vi "Flancos_3.vi"() -> ()   [LabVIEW 2017]
panel:
  out "Conteo 4":bool
  out "Conteo 3":bool
  out "Conteo 2":bool
  in  "Alarma":bool
  in  "Alarma 2":bool
  in  "Alarma 3":bool
  in  "Alarma 4":bool
  out "Conteo":bool
  in  "Seleccion":bool
  out "Waveform Chart":dbl(graph)
  out "Falling 4":dbl
  out "Rise 4":dbl
  out "Falling 3":dbl
  out "Rise 3":dbl
  out "Falling 2":dbl
  out "Rise 2":dbl
  out "Falling":dbl
  out "Rise":dbl
  in  "stop":bool
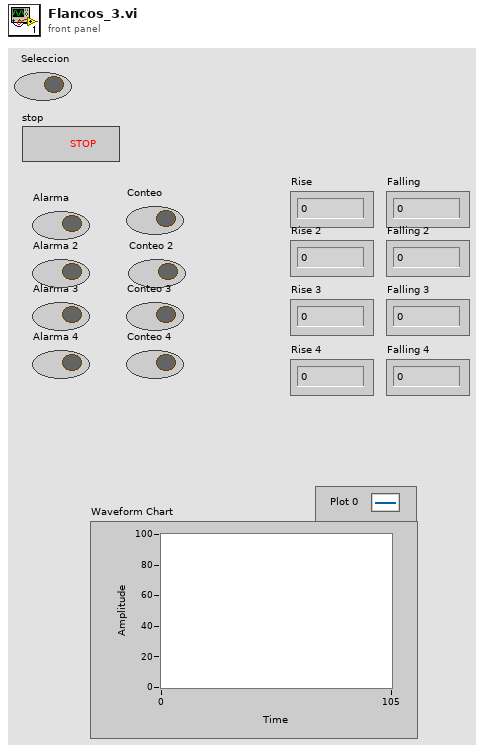
[diagram p1: front panel]
types:
  T1 = cluster{"Cont":i32, "Cont2":i32, "Cont3":i32, "Cont4":i32, "Bajada":i32, "Bajada 2":i32, "Bajada 3":i32, "Bajada 4":i32}
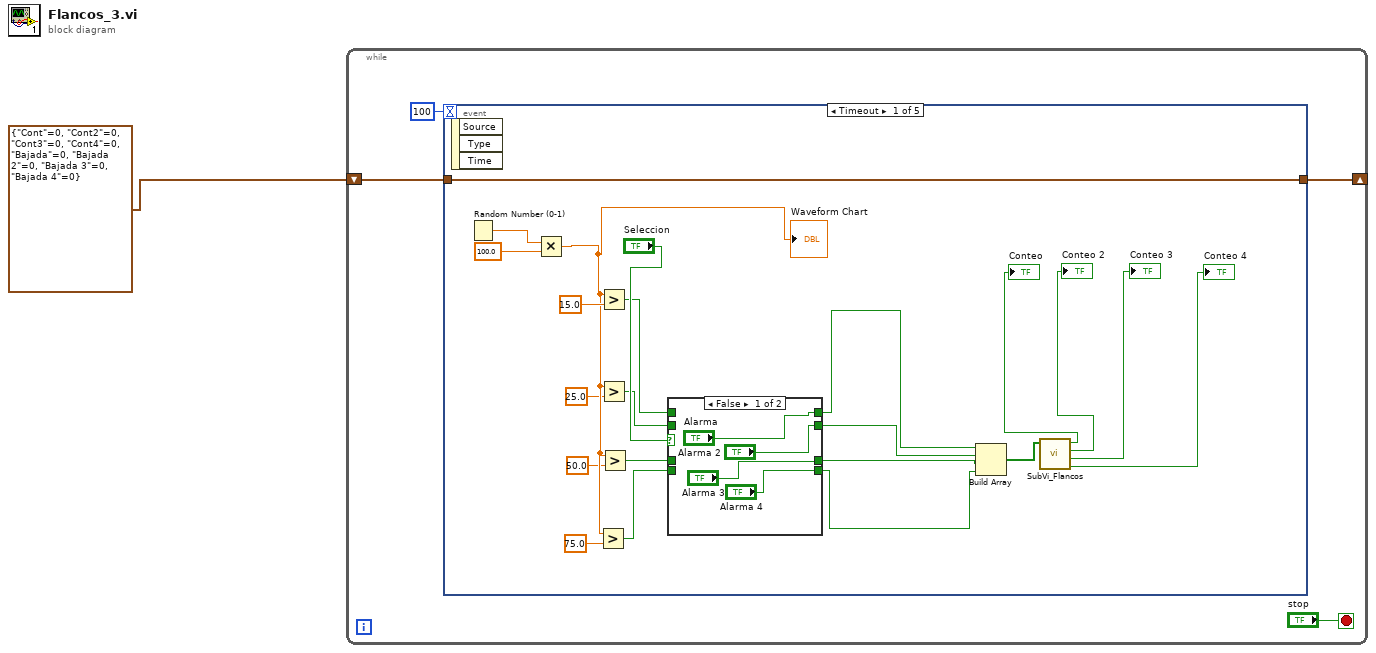
[diagram p0: block diagram]
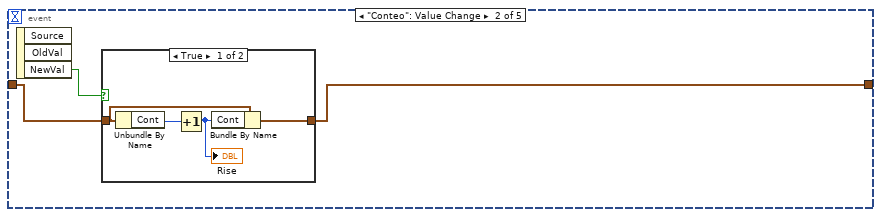
[diagram p3: hidden frame]
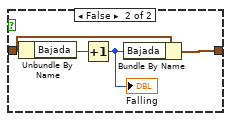
[diagram p4: hidden frame]
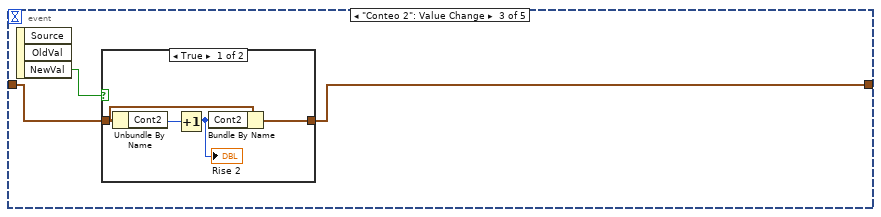
[diagram p5: hidden frame]
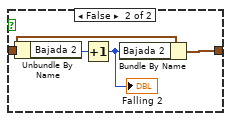
[diagram p6: hidden frame]
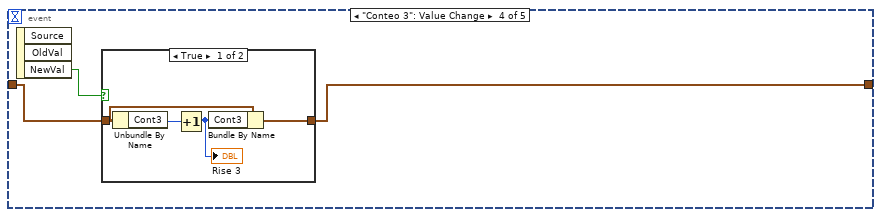
[diagram p7: hidden frame]
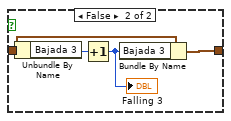
[diagram p8: hidden frame]
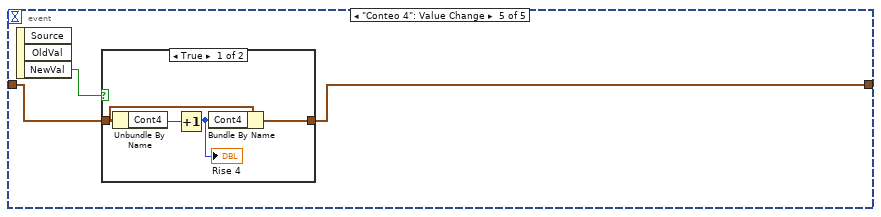
[diagram p9: hidden frame]
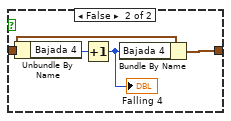
[diagram p10: hidden frame]
diagram:
  n1 = while {
    shift-right: [w3] -> _
    shift-left: T1 {"Cont"=0, "Cont2"=0, "Cont3"=0, "Cont4"=0, "Bajada"=0, "Bajada 2"=0, "Bajada 3"=0, "Bajada 4"=0} -> [w5]
    stop <- "stop" stop-if-true
    n2 = event shown="[0] Timeout" {
      selector: _ -> [_ _ _ _ _]
      dyn-events: _ -> [_ _ _ _ _]
      timeout: 100 -> [_ _ _ _ _]
      tunnel: w5 -> [w27 w38 w49 w60 w71]
      tunnel: [w27 w37 w48 w59 w70] -> w3
      event Timeout {
        n3 = event-data() -> ()  [unwired: 1 in, 3 out]
        n4 = Random Number (0-1)() -> (number: 0 to 1=w26:dbl)
        n5 = Multiply(x=w26, y=100.0) -> (x*y=w23:dbl)
        "Waveform Chart" <- w23
        n6 = Greater?(x=w23, y=75.0) -> (0:w15:bool)
        n7 = Greater?(x=w23, y=15.0) -> (0:w18:bool)
        n8 = Greater?(x=w23, y=25.0) -> (0:w17:bool)
        n9 = Greater?(x=w23, y=50.0) -> (0:w16:bool)
        n10 = case shown="False" "Seleccion" {
          tunnel: w18 -> [_ w35]
          tunnel: w17 -> [_ w34]
          tunnel: w16 -> [_ w33]
          tunnel: w15 -> [_ w32]
          tunnel: ["Alarma" w35] -> w11
          tunnel: ["Alarma 2" w34] -> w12
          tunnel: ["Alarma 3" w33] -> w13
          tunnel: ["Alarma 4" w32] -> w14
          frame False {
          }
          frame True {
          }
        }
        n11 = Build Array(w11, w12, w13, w14) -> (w10:bool[])
        n12 = call "SubVi_Flancos.vi"("Alarmas"=w10) -> ("Conteo 3"=→"Conteo 4":bool, "Conteo 2"=→"Conteo 3":bool, "Conteo 1"=→"Conteo 2":bool, "Conteo"=→"Conteo":bool)  [unwired: 7 in]
      }
      event "Conteo": Value Change {
        n13 = event-data() -> ("NewVal"=w36:bool)  [unwired: 1 in, 2 out]
        n14 = case shown="True" w36 {
          tunnel: w38 -> [w41 w45]
          tunnel: [w40 w44] -> w37
          frame True {
            n15 = Unbundle By Name(w41) -> ("Cont"=w42:i32)
            n16 = Increment(x=w42) -> (x+1=w39:i32)
            "Rise" <- w39
            n17 = Bundle By Name(cluster=w41, "Cont"=w39) -> (w40:T1)
          }
          frame False {
            n18 = Unbundle By Name(w45) -> ("Bajada"=w46:i32)
            n19 = Increment(x=w46) -> (x+1=w43:i32)
            "Falling" <- w43
            n20 = Bundle By Name(cluster=w45, "Bajada"=w43) -> (w44:T1)
          }
        }
      }
      event "Conteo 2": Value Change {
        n21 = event-data() -> ("NewVal"=w47:bool)  [unwired: 1 in, 2 out]
        n22 = case shown="True" w47 {
          tunnel: w49 -> [w52 w56]
          tunnel: [w51 w55] -> w48
          frame True {
            n23 = Unbundle By Name(w52) -> ("Cont2"=w53:i32)
            n24 = Increment(x=w53) -> (x+1=w50:i32)
            "Rise 2" <- w50
            n25 = Bundle By Name(cluster=w52, "Cont2"=w50) -> (w51:T1)
          }
          frame False {
            n26 = Unbundle By Name(w56) -> ("Bajada 2"=w57:i32)
            n27 = Increment(x=w57) -> (x+1=w54:i32)
            "Falling 2" <- w54
            n28 = Bundle By Name(cluster=w56, "Bajada 2"=w54) -> (w55:T1)
          }
        }
      }
      event "Conteo 3": Value Change {
        n29 = event-data() -> ("NewVal"=w58:bool)  [unwired: 1 in, 2 out]
        n30 = case shown="True" w58 {
          tunnel: w60 -> [w63 w67]
          tunnel: [w62 w66] -> w59
          frame True {
            n31 = Unbundle By Name(w63) -> ("Cont3"=w64:i32)
            n32 = Increment(x=w64) -> (x+1=w61:i32)
            "Rise 3" <- w61
            n33 = Bundle By Name(cluster=w63, "Cont3"=w61) -> (w62:T1)
          }
          frame False {
            n34 = Unbundle By Name(w67) -> ("Bajada 3"=w68:i32)
            n35 = Increment(x=w68) -> (x+1=w65:i32)
            "Falling 3" <- w65
            n36 = Bundle By Name(cluster=w67, "Bajada 3"=w65) -> (w66:T1)
          }
        }
      }
      event "Conteo 4": Value Change {
        n37 = event-data() -> ("NewVal"=w69:bool)  [unwired: 1 in, 2 out]
        n38 = case shown="True" w69 {
          tunnel: w71 -> [w74 w78]
          tunnel: [w73 w77] -> w70
          frame True {
            n39 = Unbundle By Name(w74) -> ("Cont4"=w75:i32)
            n40 = Increment(x=w75) -> (x+1=w72:i32)
            "Rise 4" <- w72
            n41 = Bundle By Name(cluster=w74, "Cont4"=w72) -> (w73:T1)
          }
          frame False {
            n42 = Unbundle By Name(w78) -> ("Bajada 4"=w79:i32)
            n43 = Increment(x=w79) -> (x+1=w76:i32)
            "Falling 4" <- w76
            n44 = Bundle By Name(cluster=w78, "Bajada 4"=w76) -> (w77:T1)
          }
        }
      }
    }
  }
